vi "子VI-深度学习自动检测.vi"(0 "临界Z值":i32, 1 "判定为筋条的长宽比阈值":i32, 5 "临界面积百分比值":dbl, 7 "缺陷灰度阈值":dbl caption="值", 9 "计入缺陷的面积阈值":i32, 11 "穿透图原始路径":path, 12 "计入缺陷的Z值阈值":i32 caption="值") -> (6 "全部检测结果":string[][](table))   [LabVIEW 2018]
panel:
  out "计算时间（秒）":string
  in  "stop":bool caption="停止"
  out "模型预测进度（请等待2-3分钟）":u8(slide) scale=0.0..300.0
  out "模型所在路径":path
  out "error out":errorcluster caption="错误输出"
  out "预测图片保存路径":path
  in  "选项卡控件":enum32{"原图", "预测结果", "分层类结果"}(tab)
  out "原图":T1(plugin-control)
  out "预测输出":T1(plugin-control)
  out "Threshold Image":T1(plugin-control)
  out "standard output":string
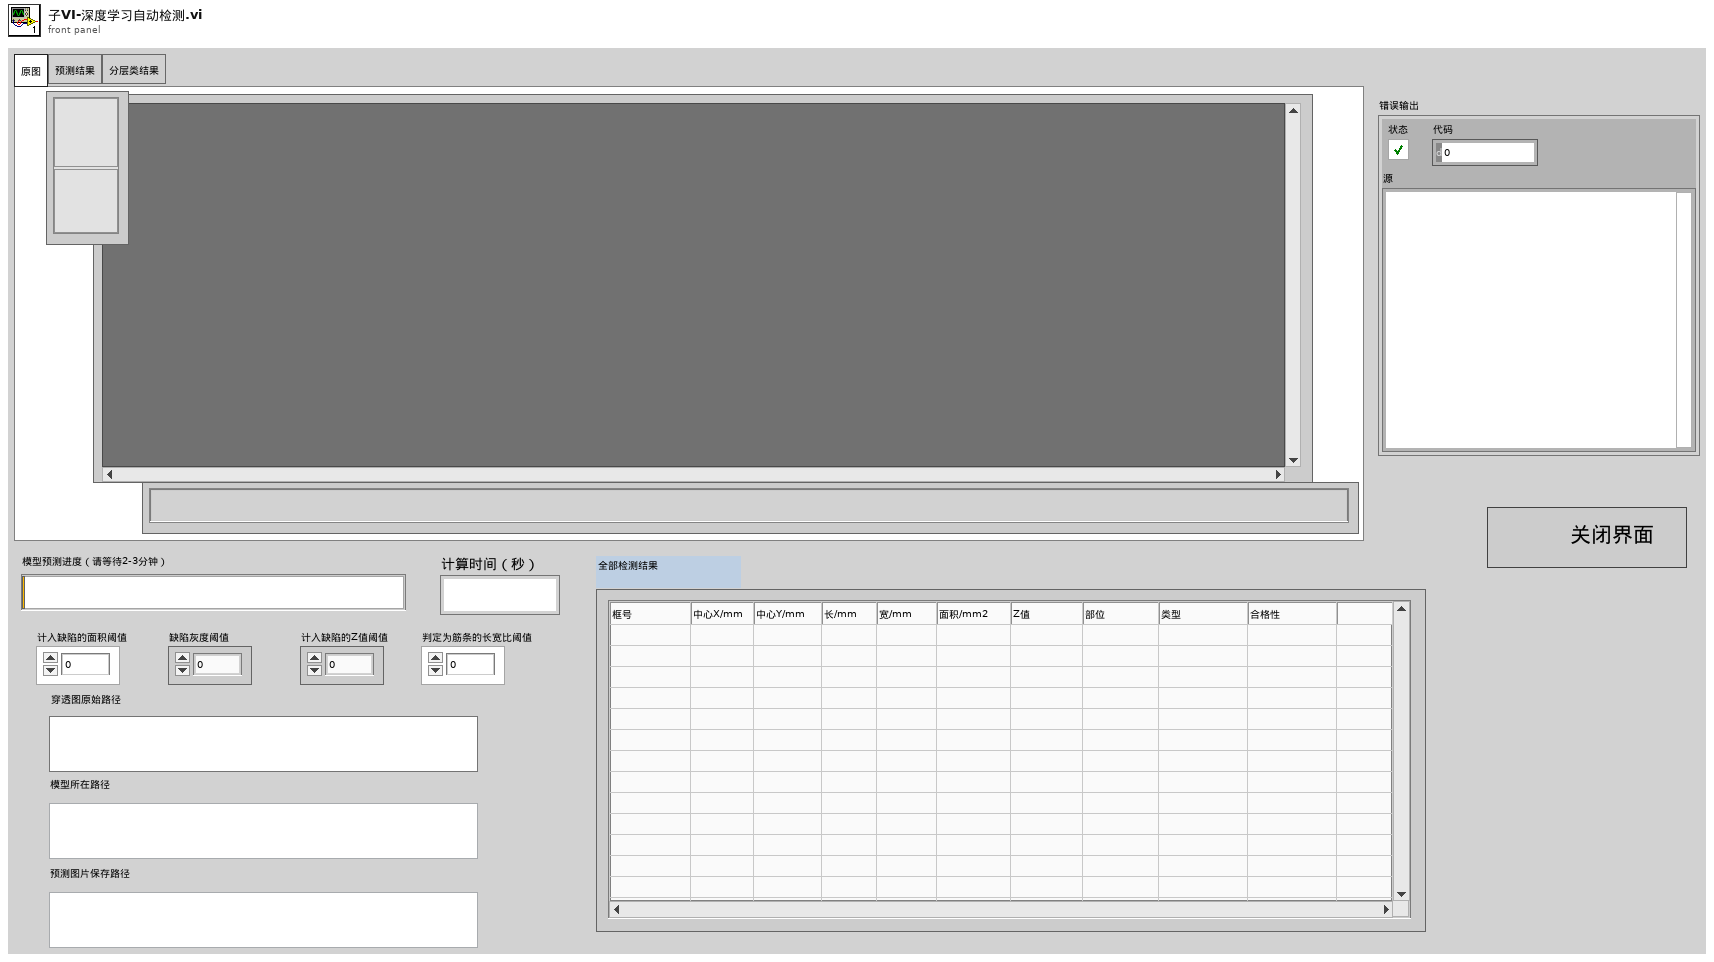
[diagram p1: front panel]
types:
  T1 = typedef "IMAQ Image.ctl" = refnum<image>
  T2 = typedef "Image Type" = u32
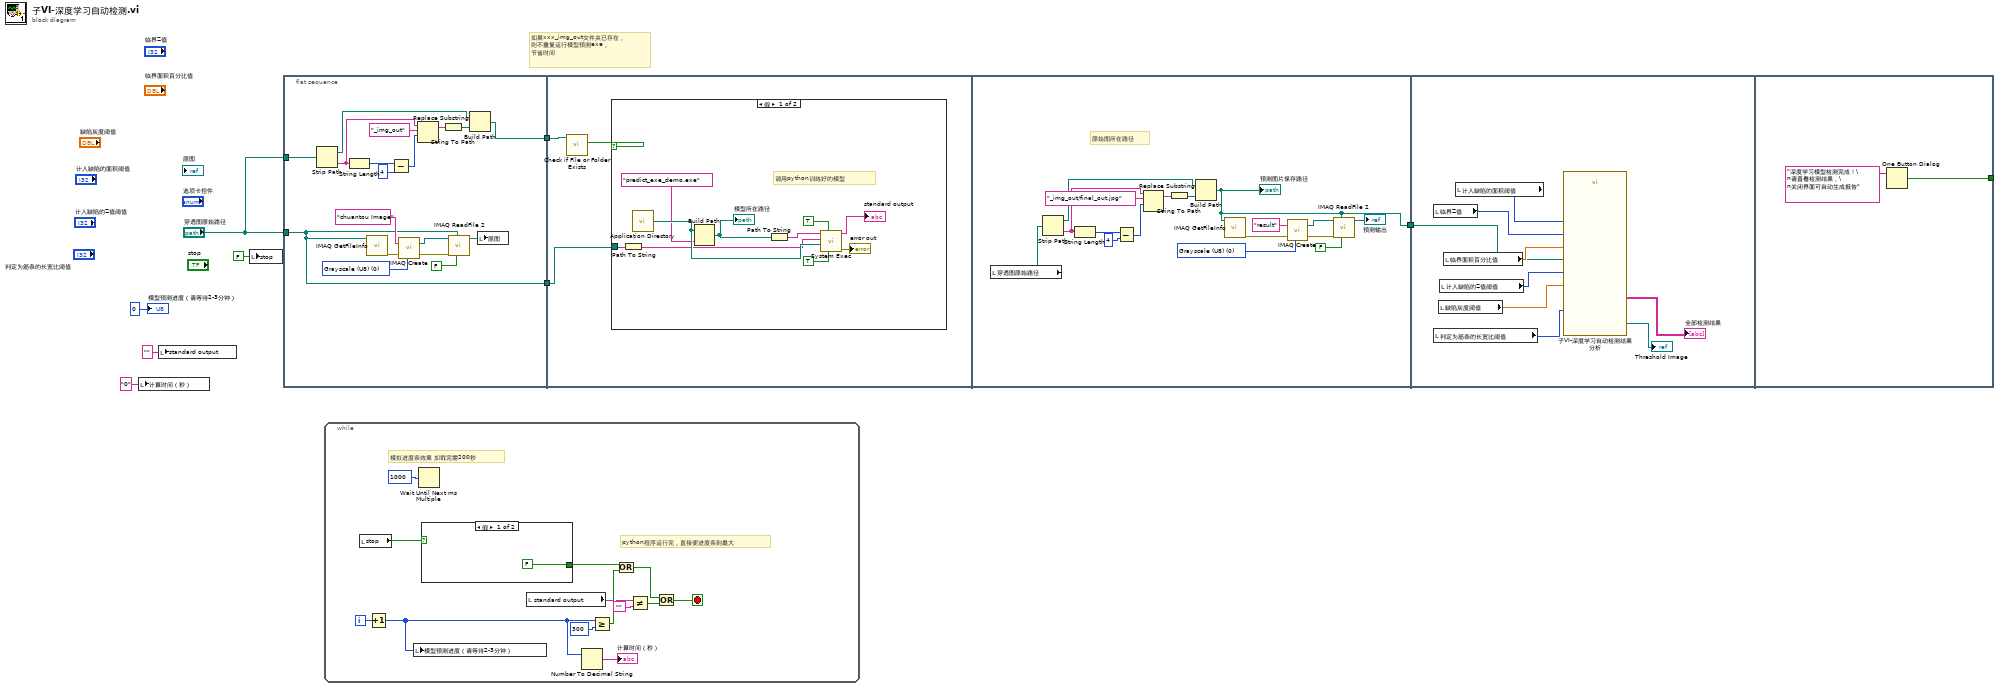
[diagram p0: block diagram]
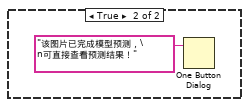
[diagram p2: hidden frame]
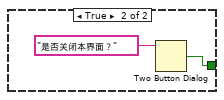
[diagram p3: hidden frame]
diagram:
  # "如果xxx_img_out文件夹已存在，\n则不重复运行模型预测exe，\n节省时间"
  n1 = local write "计算时间（秒）"("0" ("计算时间（秒）")) -> ()
  n2 = local write "standard output"("" ("standard output")) -> ()
  n3 = local write "stop"(FALSE ("stop")) -> ()
  n4 = flat-sequence {
    tunnel: [w19] -> w6
    tunnel: "穿透图原始路径" -> [w19]
    tunnel: "穿透图原始路径" -> [w10]
    tunnel: [w9] -> w2
    tunnel: w6 -> [w28]
    tunnel: w2 -> [w29]
    tunnel: [w41] -> w5
    tunnel: w5 -> [w64]
    tunnel: [w67] -> _
    frame #0 {
      w21 = T2 0 items=["Grayscale (U8)", "Grayscale (I16)", "Grayscale (SGL)", "Complex (CSG)", "RGB (U32)", "HSL (U32)", "RGB (U64)", "Grayscale (U16)"] ("Image Type")
      n5 = Strip Path(path=w10) -> (stripped path=w17:path, name=w18:string)
      n6 = String Length(string=w18) -> (length=w15:i32)
      n7 = call "IMAQ GetFileInfo"("File Path"=w19) -> ("error out"=w24:errorcluster)  [unwired: 4 in, 6 out]
      n8 = Subtract(x=w15, y=4) -> (x-y=w14:i32)
      n9 = call "IMAQ Create"("Image Name"="chuantou Image", "Image Type"=w21, "error in (no error)"=w24) -> ("New Image"=w25:T1, "error out"=w26:errorcluster)  [unwired: 2 in]
      n10 = Replace Substring(3:w14, 4:"_img_out" ("字符串"), 5:w18) -> (1:w16:string)  [unwired: 1 in, 1 out]
      n11 = String To Path(string=w16) -> (path=w13:path)
      n12 = call "IMAQ ReadFile 2"("Use File Path Image Type"=FALSE, "File Path"=w19, "error in (no error)"=w26, "Image"=w25) -> ("Image Out"=w23:T1)  [unwired: 3 in, 4 out]
      n13 = Build Path(base path=w17, name or relative path=w13) -> (appended path=w9:path)
      n14 = local write "原图"(w23) -> ()
    }
    frame #1 {
      n15 = call <vilib>:"Check if File or Folder Exists.vi"("path"=w29) -> ("file or folder exists?"=w27:bool)  [unwired: 8 in, 2 out]
      n16 = case shown="假" w27 {
        tunnel: w28 -> [w30 _]
        frame False {
          # "调用python训练好的模型"
          n17 = Path To String(path=w30) -> (string=w36:string)
          n18 = call <vilib>:"Application Directory.vi"() -> ("Application Directory"=w37:path)
          n19 = Build Path(base path=w37, name or relative path="predict_exe_demo.exe" ("名称或相对路径")) -> (appended path=w38:path)
          "模型所在路径" <- w38
          n20 = Path To String(path=w38) -> (string=w39:string)
          n21 = call <vilib>:"System Exec.vi"("run minimized? (F)"=TRUE, "wait until completion? (T)"=TRUE, "working directory"=w37, "standard input"=w36, "command line"=w39) -> ("error out"=→"error out":errorcluster, "standard output"=→"standard output":string)  [unwired: 3 in, 2 out]
        }
        frame True {
          n22 = One Button Dialog(message="该图片已完成模型预测，\n可直接查看预测结果！" ("消息")) -> ()  [unwired: 1 in, 1 out]
        }
      }
    }
    frame #2 {
      w53 = T2 0 items=["Grayscale (U8)", "Grayscale (I16)", "Grayscale (SGL)", "Complex (CSG)", "RGB (U32)", "HSL (U32)", "RGB (U64)", "Grayscale (U16)"] ("Image Type")
      # "原始图所在路径"
      n23 = local read "穿透图原始路径"() -> (w42:path)
      n24 = Strip Path(path=w42) -> (stripped path=w44:path, name=w43:string)
      n25 = String Length(string=w43) -> (length=w48:i32)
      n26 = Subtract(x=w48, y=4) -> (x-y=w49:i32)
      n27 = Replace Substring(3:w49, 4:"_img_out/final_out.jpg" ("字符串"), 5:w43) -> (1:w47:string)  [unwired: 1 in, 1 out]
      n28 = String To Path(string=w47) -> (path=w50:path)
      n29 = Build Path(base path=w44, name or relative path=w50) -> (appended path=w41:path)
      "预测图片保存路径" <- w41
      n30 = call "IMAQ GetFileInfo"("File Path"=w41) -> ("error out"=w55:errorcluster)  [unwired: 4 in, 6 out]
      n31 = call "IMAQ Create"("Image Name"="result", "Image Type"=w53, "error in (no error)"=w55) -> ("New Image"=w56:T1, "error out"=w57:errorcluster)  [unwired: 2 in]
      n32 = call "IMAQ ReadFile 2"("Use File Path Image Type"=FALSE, "File Path"=w41, "error in (no error)"=w57, "Image"=w56) -> ("Image Out"=→"预测输出":T1)  [unwired: 3 in, 4 out]
    }
    frame #3 {
      n33 = local read "临界Z值"() -> (w66:i32)
      n34 = local read "判定为筋条的长宽比阈值"() -> (w59:i32)
      n35 = local read "缺陷灰度阈值"() -> (w60:dbl)
      n36 = local read "计入缺陷的Z值阈值"() -> (w61:i32)
      n37 = local read "临界面积百分比值"() -> (w65:dbl)
      n38 = local read "计入缺陷的面积阈值"() -> (w62:i32)
      n39 = call "子VI-深度学习自动检测结果分析.vi"("计入缺陷的Z值阈值"=w61, "判定为筋条的长宽比阈值"=w59, "临界Z值"=w66, "缺陷灰度阈值"=w60, "临界面积百分比值"=w65, "计入缺陷的面积阈值"=w62, "预测图片保存路径"=w64) -> ("全部检测结果"=→"全部检测结果":string[][], 19:→"Threshold Image":T1)  [unwired: 11 in]
    }
    frame #4 {
      n40 = One Button Dialog(message="深度学习模型检测完成！\n请查看检测结果，\n关闭界面可自动生成报告" ("消息")) -> (true=w67:bool)  [unwired: 1 in]
    }
  }
  n41 = while {
    i -> [w76]
    stop <- w74 stop-if-true
    # "python程序运行完，直接使进度条到最大"
    # "模拟进度条效果 加载完需200秒"
    n42 = local read "stop"() -> (w78:bool)
    n43 = Increment(x=w76) -> (x+1=w69:i32)
    n44 = local write "模型预测进度（请等待2-3分钟）"(w69) -> ()
    n45 = Wait Until Next ms Multiple(millisecond multiple=u32 1000 ("毫秒倍数")) -> ()  [unwired: 1 out]
    n46 = case shown="假" w78 {
      tunnel: [FALSE ("T button?") w83] -> w77
      frame False {
      }
      frame True {
        n47 = Two Button Dialog(message="是否关闭本界面？" ("消息")) -> (T button?=w83:bool)  [unwired: 2 in]
      }
    }
    n48 = local read "standard output"() -> (w73:string)
    n49 = Number To Decimal String(number=w69) -> (decimal integer string=→"计算时间（秒）":string)  [unwired: 1 in]
    n50 = Greater Or Equal?(x=w69, y=300) -> (x >= y?=w79:bool)
    n51 = Or(x=w77, y=w79) -> (x .or. y?=w75:bool)
    n52 = Not Equal?(x=w73, y="") -> (x != y?=w71:bool)
    n53 = Or(x=w75, y=w71) -> (x .or. y?=w74:bool)
  }
  "模型预测进度（请等待2-3分钟）" <- u8 0 ("模型运行进度")
